vi "Random_Number.vi"() -> ()   [LabVIEW 2020]
panel:
  out "Output":dbl format="%#_13g"
  out "Random Number":dbl format="%#_13g"
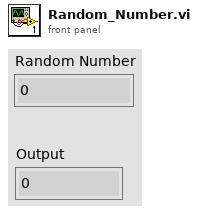
[diagram p1: front panel]
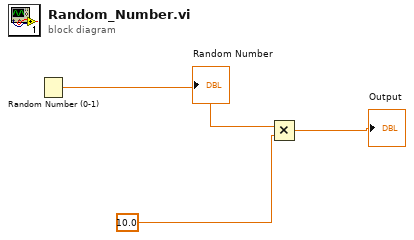
[diagram p0: block diagram]
diagram:
  n1 = Random Number (0-1)() -> (number: 0 to 1=w3:dbl)
  "Random Number" <- w3
  n2 = Multiply(x=w3, y=10.0 ("Units\nUnits")) -> (x*y=→"Output":dbl)
